vi "Format HW label name.vi"(8 "formatting":enum16{"NIVeriStandAdd-Ons", "ni"}(ring), 9 "Label Name in":string, 10 "SDI":i32, 11 "Label Decimal":i32) -> (3 "Label Name out":string)   [LabVIEW 2020]
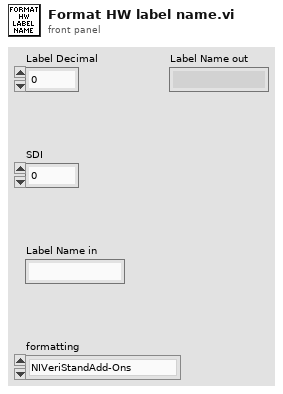
[diagram p1: front panel]
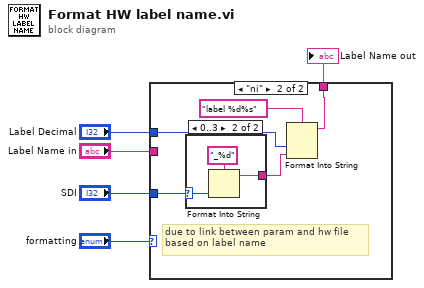
[diagram p0: block diagram]
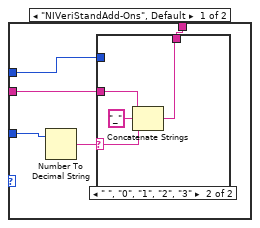
[diagram p2: hidden frame]
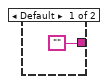
[diagram p4: hidden frame]
diagram:
  n1 = case shown="\"ni\"" "formatting" {
    tunnel: [w10 w18] -> w1
    tunnel: "Label Name in" -> [w8 _]
    tunnel: "SDI" -> [w7 w17]
    tunnel: "Label Decimal" -> [w6 w19]
    frame "NIVeriStandAdd-Ons", Default {
      n2 = Number To Decimal String(number=w7) -> (decimal integer string=w9:string)  [unwired: 1 in]
      n3 = case shown="\" \", \"0\", \"1\", \"2\", \"3\"" w9 {
        selector: w9 -> [_ w12]
        tunnel: w8 -> [w11 w15]
        tunnel: [w11 w13] -> w10
        tunnel: w6 -> [_ _]
        frame "False", Default {
        }
        frame " ", "0", "1", "2", "3" {
          n4 = Concatenate Strings(w15, "_" ("string"), w12) -> (w13:string)
        }
      }
    }
    frame "ni" {
      # "due to link between param and hw file\nbased on label name"
      n5 = case shown="0..3" w17 {
        selector: w17 -> [_ w23]
        tunnel: ["" w22] -> w16
        frame Default {
        }
        frame 0..3 {
          n6 = Format Into String(format string="_%d", w23) -> (resulting string=w22:string)  [unwired: 2 in, 1 out]
        }
      }
      n7 = Format Into String(format string="label %d%s", w19, w16) -> (resulting string=w18:string)  [unwired: 2 in, 1 out]
    }
  }
  "Label Name out" <- w1
